vi "Test Single Execution of Experimental Driver.vi"() -> (0 "Reason":string, 1 "Success":bool)   [LabVIEW 2013]
uses:
  <vilib>/xml/Load XML File.vi
  <vilib>/xml/NI_XML.lvlib
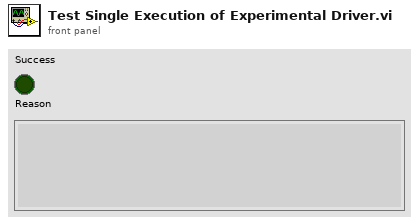
[diagram p1: front panel]
types:
  T1 = typedef "Sidecar Debug Queue.ctl" = refnum<queue>
  T2 = typedef "Experimental Configuration.ctl" = cluster{"Output Waveforms":waveform(dbl)[], "Output Channels":string, "Input Channels":string, "Post-Hook Occurence":refnum<k4>}
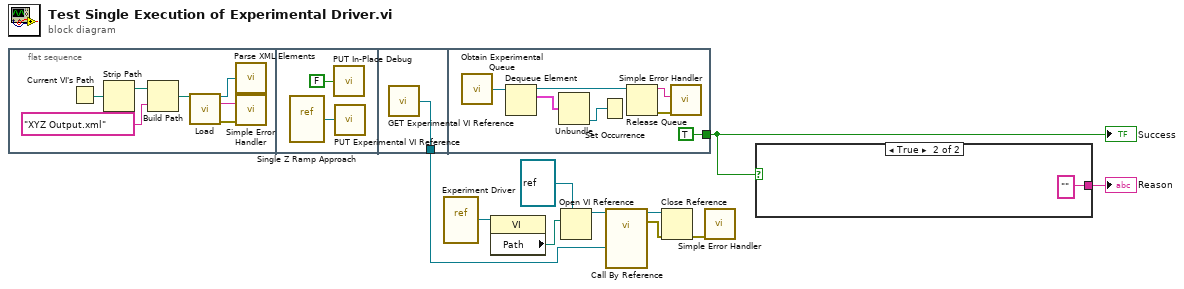
[diagram p0: block diagram]
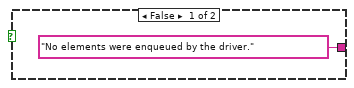
[diagram p2: hidden frame]
diagram:
  n1 = flat-sequence {
    tunnel: [w20] -> w3
    tunnel: [TRUE] -> w1
    frame #0 {
      n2 = Current VI's Path() -> (path=w17:path)
      n3 = Strip Path(path=w17) -> (stripped path=w16:path)  [unwired: 1 out]
      n4 = Build Path(base path=w16, name or relative path="XYZ Output.xml") -> (appended path=w11:path)
      n5 = call-poly <vilib>:"Load.vi"("path to XML document"=w11) -> ("DOM document out"=w14:refnum<k20>, "parse errors"=w12:string, "error out"=w13:errorcluster)  [unwired: 12 in]
      n6 = call "Parse XML Elements.vi"("DOM"=w14) -> ()
      n7 = call <vilib>:"Simple Error Handler.vi"("error source (\" \")"=w12, "error in (no error)"=w13) -> ()  [unwired: 3 in, 5 out]
    }
    frame #1 {
      n8 = vi-ref "Single Z Ramp Approach.vi"() -> (w18:refnum<vi>)
      n9 = call "PUT In-Place Debug.vi"("In Place Debug Enabled"=FALSE) -> ()
      n10 = call "PUT Experimental VI Reference.vi"("Experimental VI Reference"=w18) -> ()
    }
    frame #2 {
      n11 = call "GET Experimental VI Reference.vi"() -> ("Experimental VI Reference"=w20:refnum<vi>)
    }
    frame #3 {
      n12 = call "Obtain Experimental Queue.vi"() -> ("Queue"=w24:T1)
      n13 = Dequeue Element(queue=w24) -> (queue out=w25:T1, element=w23:T2)  [unwired: 2 in, 2 out]
      n14 = Unbundle(w23) -> ("Post-Hook Occurence"=w22:refnum<k4>)  [unwired: 3 out]
      n15 = Set Occurrence(w22) -> ()
      n16 = Release Queue(queue=w25) -> (queue name=w26:string, error out=w27:errorcluster)  [unwired: 2 in, 1 out]
      n17 = call <vilib>:"Simple Error Handler.vi"("error source (\" \")"=w26, "error in (no error)"=w27) -> ()  [unwired: 3 in, 5 out]
    }
  }
  n18 = vi-ref "Experiment Driver.vi"() -> (w4:refnum<vi>)
  n19 = property class="VI"(reference=w4) -> ("Path"=w6:path)  [unwired: 1 in, 2 out]
  n20 = Open VI Reference(type specifier VI Refnum (for type only)=refnum<vi> refnum, vi path=w6) -> (vi reference=w7:refnum<vi>)  [unwired: 4 in, 1 out]
  n21 = call-by-ref "?"(reference=w7, "Experiment VI Reference"=w3) -> (reference out=w8:refnum<vi>, error out=w9:errorcluster)  [unwired: 1 in]
  n22 = Close Reference(reference=w8, error in (no error)=w9) -> (error out=w2:errorcluster)
  n23 = call <vilib>:"Simple Error Handler.vi"("error in (no error)"=w2) -> ()  [unwired: 4 in, 5 out]
  n24 = case shown="True" w1 {
    tunnel: ["No elements were enqueued by the driver." ("name or relative path") "" ("name or relative path")] -> w10
    frame False {
    }
    frame True {
    }
  }
  "Reason" <- w10
  "Success" <- w1
